vi "Main - Time to Seconds (SubVI).vi"(7 "String?":bool, 10 "Time String":string, 11 "Time":timestamp format="%<%H:%M:%S>T") -> (3 "Seconds":dbl)   [LabVIEW 2019]
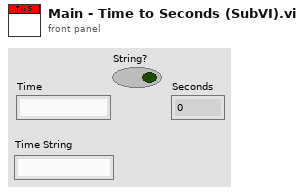
[diagram p1: front panel]
types:
  T1 = typedef "LVDateTimeRec.ctl" = cluster{"fractional second":dbl, "second":i32, "minute":i32, "hour":i32, "day of month":i32, "month":i32, "year":i32, "day of week":i32, "day of year":i32, "DST":i32}
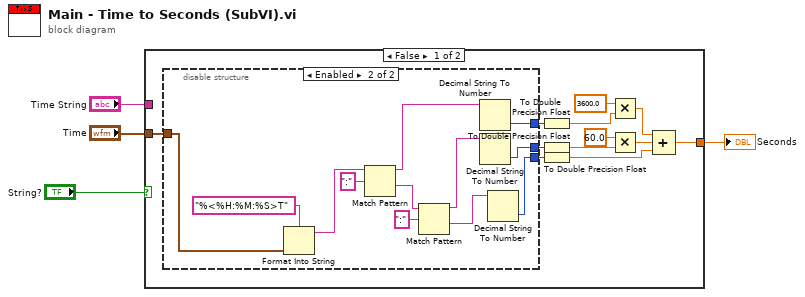
[diagram p0: block diagram]
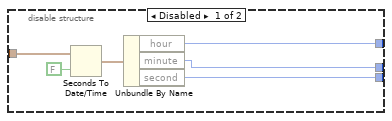
[diagram p2: hidden frame]
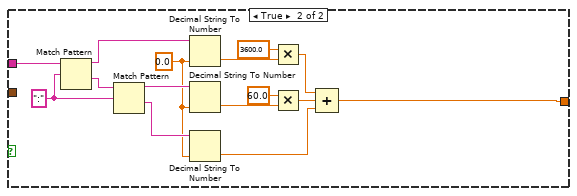
[diagram p3: hidden frame]
diagram:
  n1 = case shown="False" "String?" {
    tunnel: [w16 w35] -> w4
    tunnel: "Time" -> [w15 _]
    tunnel: "Time String" -> [_ w49]
    frame False {
      n2 = disable-structure shown="Enabled" {
        disable-tunnel: w15 -> [w22 w26]
        disable-tunnel: [w20 w23] -> w11
        disable-tunnel: [w19 w24] -> w8
        disable-tunnel: [w18 w25] -> w5
        frame Disabled {
          n3 = Seconds To Date/Time(time stamp (now)=w22, to UTC (F)=FALSE) -> (date time rec=w17:T1)
          n4 = Unbundle By Name(w17) -> ("hour"=w18:i32, "minute"=w19:i32, "second"=w20:i32)
        }
        frame Enabled {
          n5 = Format Into String(format string="%<%H:%M:%S>T", w26) -> (resulting string=w30:string)  [unwired: 2 in, 1 out]
          n6 = Match Pattern(string=w30, regular expression=":") -> (before substring=w32:string, after substring=w31:string)  [unwired: 1 in, 2 out]
          n7 = Match Pattern(string=w31, regular expression=":") -> (before substring=w33:string, after substring=w34:string)  [unwired: 1 in, 2 out]
          n8 = Decimal String To Number(string=w32) -> (number=w25:i32)  [unwired: 2 in, 1 out]
          n9 = Decimal String To Number(string=w33) -> (number=w24:i32)  [unwired: 2 in, 1 out]
          n10 = Decimal String To Number(string=w34) -> (number=w23:i32)  [unwired: 2 in, 1 out]
        }
      }
      n11 = To Double Precision Float(number=w5) -> (double precision float=w12:dbl)
      n12 = To Double Precision Float(number=w8) -> (double precision float=w13:dbl)
      n13 = To Double Precision Float(number=w11) -> (double precision float=w14:dbl)
      n14 = Multiply(x=3600.0, y=w12) -> (x*y=w9:dbl)
      n15 = Multiply(x=60.0, y=w13) -> (x*y=w10:dbl)
      n16 = Compound Arithmetic op=ADD(w9, w10, w14) -> (w16:dbl)
    }
    frame True {
      w43 = 0.0 ("default (0 I32)")
      w47 = ":" ("regular expression")
      n17 = Match Pattern(string=w49, regular expression=w47) -> (before substring=w46:string, after substring=w48:string)  [unwired: 1 in, 2 out]
      n18 = Match Pattern(string=w48, regular expression=w47) -> (before substring=w45:string, after substring=w44:string)  [unwired: 1 in, 2 out]
      n19 = Decimal String To Number(string=w46, default (0L)=w43) -> (number=w38:dbl)  [unwired: 1 in, 1 out]
      n20 = Decimal String To Number(string=w45, default (0L)=w43) -> (number=w37:dbl)  [unwired: 1 in, 1 out]
      n21 = Decimal String To Number(string=w44, default (0L)=w43) -> (number=w36:dbl)  [unwired: 1 in, 1 out]
      n22 = Multiply(x=3600.0, y=w38) -> (x*y=w41:dbl)
      n23 = Multiply(x=60.0, y=w37) -> (x*y=w42:dbl)
      n24 = Compound Arithmetic op=ADD(w41, w42, w36) -> (w35:dbl)
    }
  }
  "Seconds" <- w4
